vi "Init Thermocouples.vi"() -> (4 "task out":refnum<k21>, 15 "Error Out":errorcluster)   [LabVIEW 2018]
uses:
  <vilib>/DAQmx/create/channels.llb/DAQmx Create Channel (AI-Temperature-Thermocouple).vi
  <vilib>/DAQmx/configure/timing.llb/DAQmx Timing (Sample Clock).vi
  <resource>/objmgr/daqmx.rc
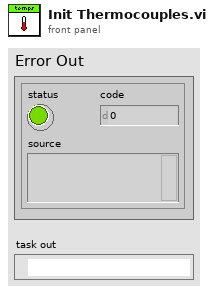
[diagram p1: front panel]
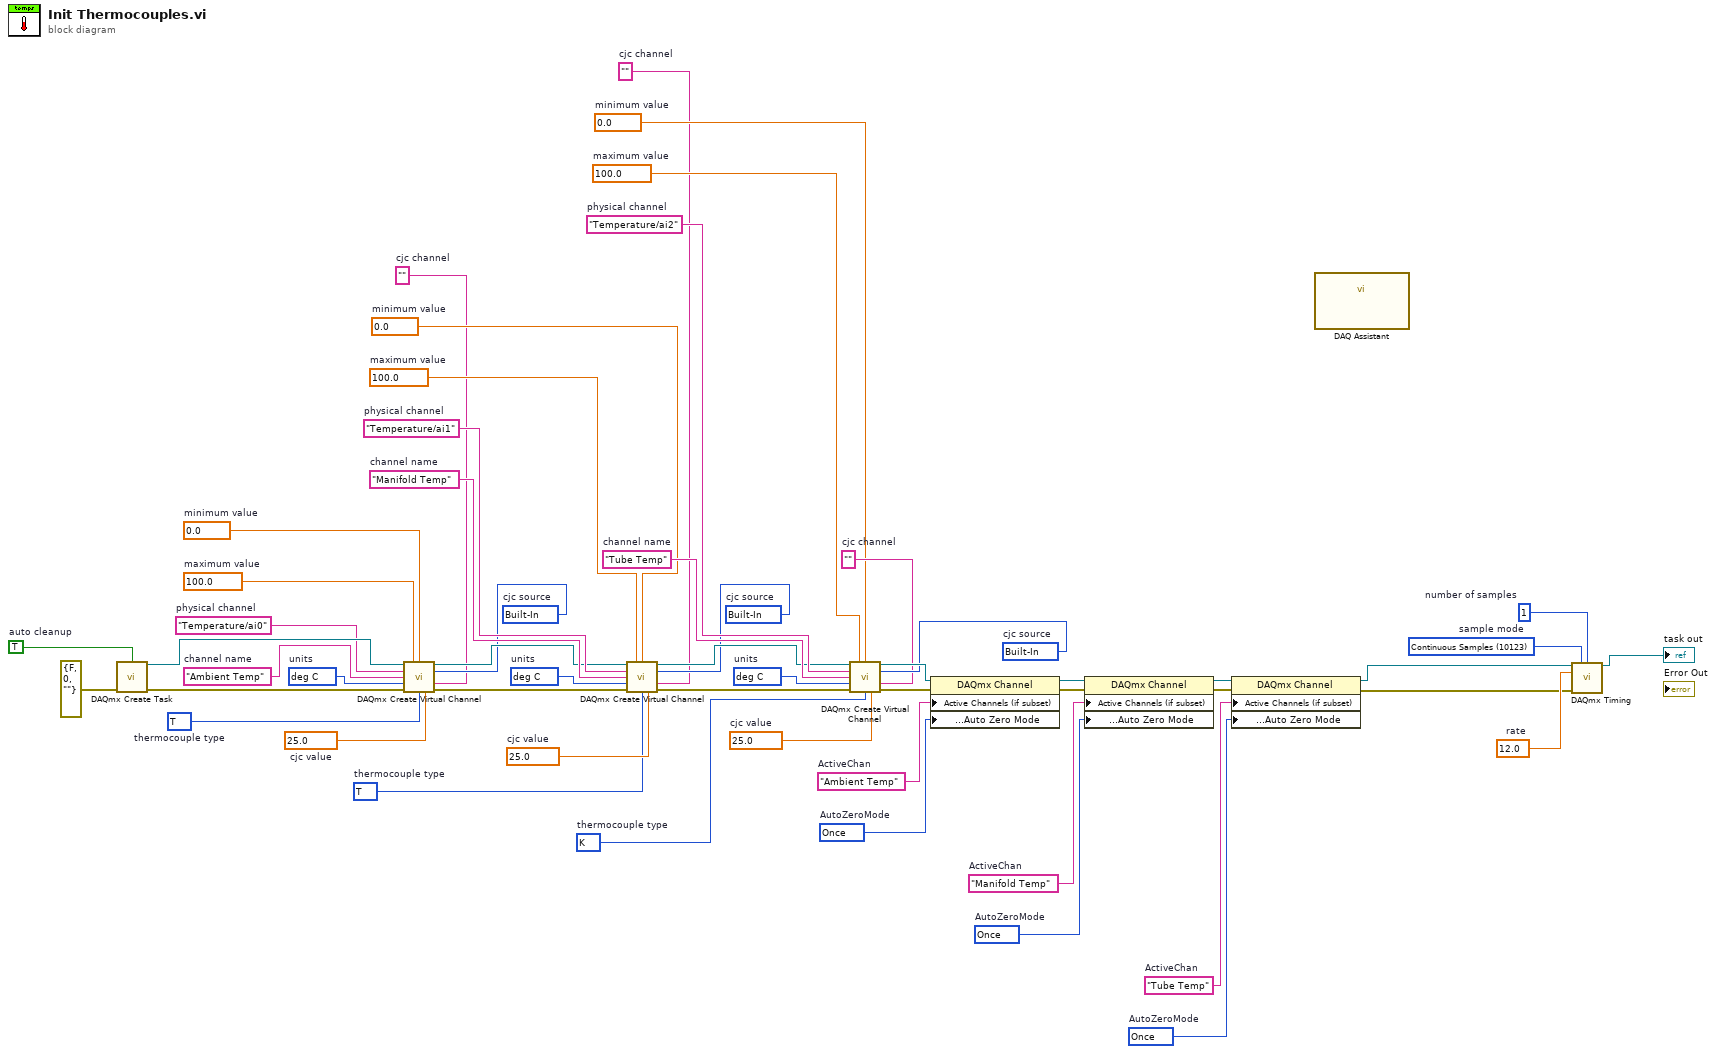
[diagram p0: block diagram]
diagram:
  w4 = 10123 items=["Finite Samples"=10178, "Continuous Samples"=10123, "Hardware Timed Single Point"=12522]  # sample mode
  w5 = 1  # number of samples
  w6 = 12.0  # rate
  w47 = 10244 items=["None"=10230, "Once"=10244, "Every Sample"=10164]  # AutoZeroMode
  w48 = "Tube Temp"  # ActiveChan
  w43 = 10244 items=["None"=10230, "Once"=10244, "Every Sample"=10164]  # AutoZeroMode
  w44 = "Manifold Temp"  # ActiveChan
  w39 = 10244 items=["None"=10230, "Once"=10244, "Every Sample"=10164]  # AutoZeroMode
  w40 = "Ambient Temp"  # ActiveChan
  w38 = 10200 items=["Built-In"=10200, "Constant Value"=10116, "Channel"=10113]  # cjc source
  w36 = ""  # cjc channel
  w35 = 25.0  # cjc value
  w34 = 10073 items=["J"=10072, "K"=10073, "N"=10077, "R"=10082, "S"=10085, "T"=10086, "B"=10047, "E"=10055]  # thermocouple type
  w33 = 10143 items=["deg C"=10143, "deg F"=10144, "Kelvins"=10325, "deg R"=10145, "From Custom Scale"=10065]  # units
  w37 = "Tube Temp"  # channel name
  w31 = 0.0  # minimum value
  w30 = 100.0  # maximum value
  w29 = "Temperature/ai2"  # physical channel
  w27 = 10200 items=["Built-In"=10200, "Constant Value"=10116, "Channel"=10113]  # cjc source
  w25 = ""  # cjc channel
  w24 = 25.0  # cjc value
  w23 = 10086 items=["J"=10072, "K"=10073, "N"=10077, "R"=10082, "S"=10085, "T"=10086, "B"=10047, "E"=10055]  # thermocouple type
  w22 = 10143 items=["deg C"=10143, "deg F"=10144, "Kelvins"=10325, "deg R"=10145, "From Custom Scale"=10065]  # units
  w26 = "Manifold Temp"  # channel name
  w20 = 0.0  # minimum value
  w19 = 100.0  # maximum value
  w18 = "Temperature/ai1"  # physical channel
  w16 = 10200 items=["Built-In"=10200, "Constant Value"=10116, "Channel"=10113]  # cjc source
  w14 = ""  # cjc channel
  w13 = 25.0  # cjc value
  w12 = 10086 items=["J"=10072, "K"=10073, "N"=10077, "R"=10082, "S"=10085, "T"=10086, "B"=10047, "E"=10055]  # thermocouple type
  w11 = 10143 items=["deg C"=10143, "deg F"=10144, "Kelvins"=10325, "deg R"=10145, "From Custom Scale"=10065]  # units
  w15 = "Ambient Temp"  # channel name
  w9 = 0.0  # minimum value
  w8 = 100.0  # maximum value
  w7 = "Temperature/ai0"  # physical channel
  w53 = TRUE  # auto cleanup
  n1 = call <vilib>:"DAQmx Create Task.vi"("auto cleanup"=w53, "error in"=errorcluster {"status"=FALSE, "code"=0, "source"=""}) -> ("task out"=w51:refnum<k21>, "error out"=w50:errorcluster)  [unwired: 12 in]
  n2 = call-poly <vilib>:"DAQmx Create Virtual Channel.vi"("task in"=w51, "maximum value"=w8, "minimum value"=w9, "physical channels"=w7, "cjc source"=w16, "name to assign"=w15, "units"=w11, "cjc channel"=w14, "error in"=w50, "thermocouple type"=w12, "cjc value"=w13) -> ("task out"=w17:refnum<k21>, "error out"=w10:errorcluster)  [unwired: 3 in]
  n3 = call-poly <vilib>:"DAQmx Create Virtual Channel.vi"("task in"=w17, "maximum value"=w19, "minimum value"=w20, "physical channels"=w18, "cjc source"=w27, "name to assign"=w26, "units"=w22, "cjc channel"=w25, "error in"=w10, "thermocouple type"=w23, "cjc value"=w24) -> ("task out"=w28:refnum<k21>, "error out"=w21:errorcluster)  [unwired: 3 in]
  n4 = call-poly <vilib>:"DAQmx Create Virtual Channel.vi"("task in"=w28, "maximum value"=w30, "minimum value"=w31, "physical channels"=w29, "cjc source"=w38, "name to assign"=w37, "units"=w33, "cjc channel"=w36, "error in"=w21, "thermocouple type"=w34, "cjc value"=w35) -> ("task out"=w41:refnum<k21>, "error out"=w32:errorcluster)  [unwired: 3 in]
  n5 = property class="DAQmx Channel"(reference=w41, error in=w32, "Active Channels (if subset)"=w40, "Analog Input:General Properties:Advanced:High Accuracy Settings:Auto Zero Mode"=w39) -> (reference out=w45:refnum<k21>, error out=w42:errorcluster)
  n6 = property class="DAQmx Channel"(reference=w45, error in=w42, "Active Channels (if subset)"=w44, "Analog Input:General Properties:Advanced:High Accuracy Settings:Auto Zero Mode"=w43) -> (reference out=w49:refnum<k21>, error out=w46:errorcluster)
  n7 = property class="DAQmx Channel"(reference=w49, error in=w46, "Active Channels (if subset)"=w48, "Analog Input:General Properties:Advanced:High Accuracy Settings:Auto Zero Mode"=w47) -> (reference out=w2:refnum<k21>, error out=w3:errorcluster)
  n8 = call "DAQ Assistant"() -> ()  [unwired: 12 in]
  n9 = call-poly <vilib>:"DAQmx Timing.vi"("task/channels in"=w2, "sample mode"=w4, "samples per channel"=w5, "rate"=w6, "error in"=w3) -> ("task out"=→"task out":refnum<k21>)  [unwired: 9 in, 1 out]
